vi "Post-Build Action.vi"(5 "Files Generated by Build":path[](array[path]), 6 "Top Level/Always Included VIs":path[](array[path]), 7 "Destination Path":path, 8 "error in (no error)":errorcluster, 9 "Target Name":string, 10 "Build Specification Name":string, 11 "Project Path":path) -> (0 "error out":errorcluster)   [LabVIEW 2027]
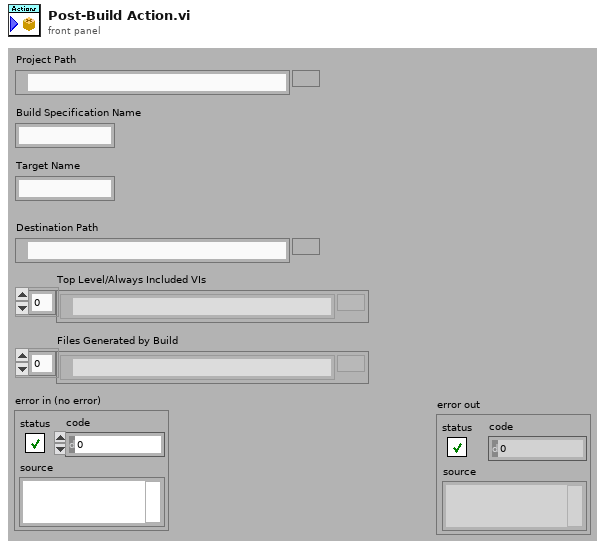
[diagram p1: front panel]
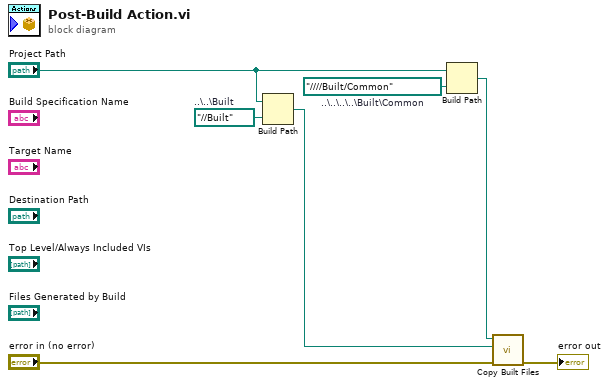
[diagram p0: block diagram]
diagram:
  w6 = path "../../../../Built/Common"  # ..\..\..\..\Built\Common
  w5 = path "../../Built"  # ..\..\Built
  n1 = Build Path(base path="Project Path", name or relative path=w5) -> (appended path=w3:path)
  n2 = Build Path(base path="Project Path", name or relative path=w6) -> (appended path=w2:path)
  n3 = call "Copy Built Files.vi"("error in (no error)"="error in (no error)", "Component Built Path"=w3, "Repo Built Path"=w2) -> ("error out"=→"error out":errorcluster)  [unwired: 8 in]
